vi "IPS Examine Status.vi"(4 "Error In":errorcluster={"status"=FALSE, "code"=1073676294, "source"="VISA Read in Prologix USB GPIB Command.vi"}, 7 "VISA resource name 2":refnum<visa-resource-name>="COM3") -> (0 "Error Out":errorcluster={"status"=FALSE, "code"=1073676294, "source"="VISA Read in Prologix_GPIB_Sample.vi"}, 1 "X Strings":T1, 2 "X Cluster":T2={"System 1"=enum."Normal", "System 2"=enum."Outside Positive Current Limi", "Activity"=enum."Hold", "Switch Heater"=enum."No Switch Fitted", "Mode 1"=enum."Amps Fast", "Mode 2"=enum."At Rest"}, 3 "VISA resource name":refnum<visa-resource-name>="GPIB1::25::INSTR")   [LabVIEW 2016, in "IPS-120.lvlib"]
uses:
  IPS-120.lvlib
  Typedefs/Read X - Cluster.ctl
  Typedefs/Read System 1 - Enum.ctl
  Typedefs/Read System 2 - Enum.ctl
  Typedefs/Read Activity - Enum.ctl
  Typedefs/Read Switch Heater - Enum.ctl
  Typedefs/Read Mode 1 - Enum.ctl
  Typedefs/Read Mode 2 - Enum.ctl
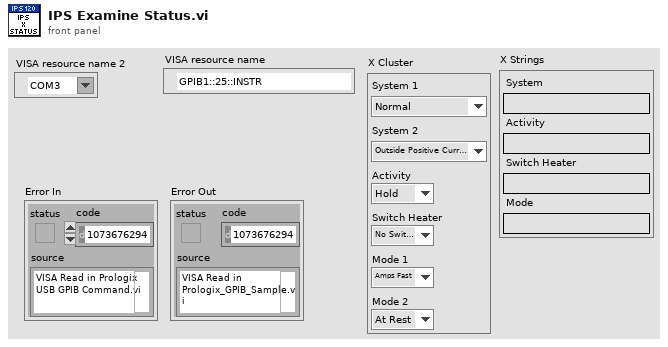
[diagram p1: front panel]
types:
  T1 = cluster{"System":string, "Activity":string, "Switch Heater":string, "Mode":string}
  T2 = typedef "IPS-120.lvlib/Read X - Cluster.ctl" = cluster{"System 1":T3, "System 2":T4, "Activity":T5, "Switch Heater":T6, "Mode 1":T7, "Mode 2":T8}
  T3 = typedef "IPS-120.lvlib/Read System 1 - Enum.ctl" = enum16{"Normal", "Quenched", "Over Heated", "Warming Up", "Fault"}
  T4 = typedef "IPS-120.lvlib/Read System 2 - Enum.ctl" = enum16{"Normal", "On Positive Voltage Limit", "On Negative Voltage Limit", "Outside Negative Current Limit", "Outside Positive Current Limi"}
  T5 = typedef "IPS-120.lvlib/Read Activity - Enum.ctl" = enum16{"Hold", "To Set Point", "To Zero", "Clamped"}
  T6 = typedef "IPS-120.lvlib/Read Switch Heater - Enum.ctl" = enum16{"Off Magnet at Zero", "On", "Off Magnet at Field", "Heater Fault", "No Switch Fitted"}
  T7 = typedef "IPS-120.lvlib/Read Mode 1 - Enum.ctl" = enum16{"Amps Fast", "Tesla Fast", "Amps Slow", "Tesla Slow"}
  T8 = typedef "IPS-120.lvlib/Read Mode 2 - Enum.ctl" = enum16{"At Rest", "Sweeping", "Sweep Limiting", "Sweeping & Sweep Limiting"}
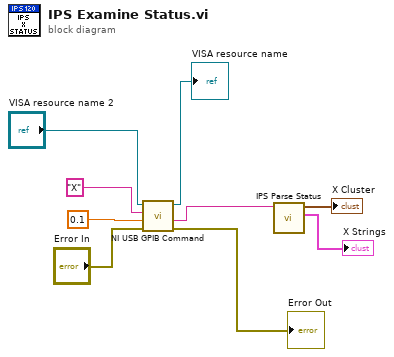
[diagram p0: block diagram]
diagram:
  n1 = call "NI USB GPIB Command.vi"("Error In"="Error In", "Wait for instrument to respond (s)"=0.1, "String to Send"="X", "VISA resource name"="VISA resource name 2") -> ("Error Out"=→"Error Out":errorcluster, "Return String from Device (Not all commands return a String)"=w3:string, "VISA resource name out"=→"VISA resource name":refnum<visa-resource-name>)  [unwired: 1 out]
  n2 = call "IPS Parse Status.vi"("X String"=w3) -> ("X Strings"=→"X Strings":T1, "X Cluster"=→"X Cluster":T2)  [unwired: 5 in]
